vi "GetUIRef.vi"(8 "error in (no error)":errorcluster, 11 "View in":refnum<class "View.lvclass">) -> (0 "error out":errorcluster, 2 "UIRef":refnum<vi>, 3 "View out":refnum<class "View.lvclass">)   [LabVIEW 2020, in "Page1.lvlib" / "View.lvclass"]
uses:
  View.lvclass
  UI.vi
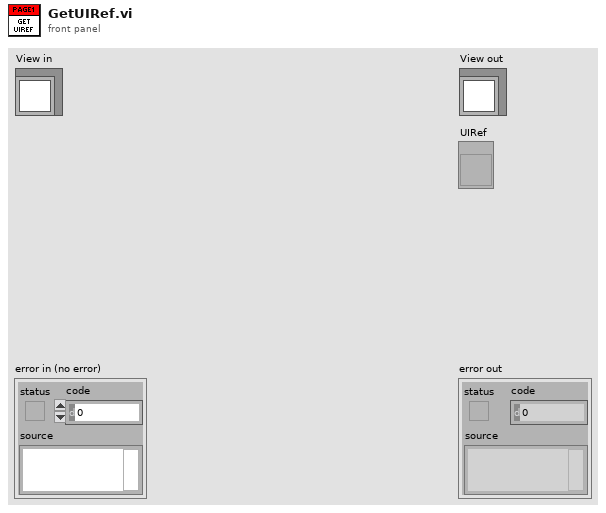
[diagram p1: front panel]
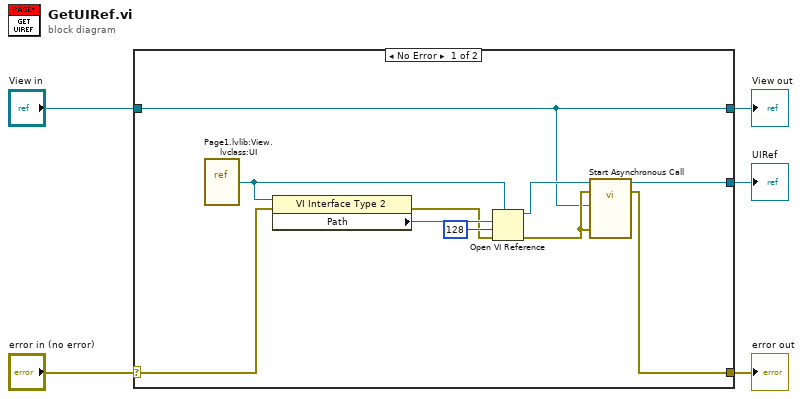
[diagram p0: block diagram]
diagram:
  n1 = case shown="No Error" "error in (no error)" {
    selector: "error in (no error)" -> [w8 w17]
    tunnel: [w14 w17] -> w4
    tunnel: [w6 w16] -> w2
    tunnel: "View in" -> [w6 w16]
    tunnel: [w15 _] -> w1
    frame No Error {
      n2 = vi-ref "Page1.lvlib:View.lvclass:UI.vi"() -> (w10:refnum<vi>)
      n3 = property class="VI Interface Type 2"(reference=w10, error in=w8) -> (error out=w9:errorcluster, "Path"=w13:path)  [unwired: 1 out]
      n4 = Open VI Reference(type specifier VI Refnum (for type only)=w10, vi path=w13, options=128, error in (no error)=w9) -> (vi reference=w11:refnum<vi>, error out=w7:errorcluster)  [unwired: 2 in]
      n5 = call-by-ref "Start Asynchronous Call"(reference=w11, error in=w7, 8:"error in (no error)"=w7, "View in"=w6) -> (reference out=w15:refnum<vi>, error out=w14:errorcluster)  [unwired: 8 in, 2 out]
    }
    frame Error {
    }
  }
  "error out" <- w4
  "View out" <- w2
  "UIRef" <- w1
